vi "ControlGenerator_Main.vi"() -> ()   [LabVIEW 2014]
uses:
  <vilib>/LabVIEW Icon API/LabVIEW Icon API.lvlib
  <vilib>/LabVIEW Icon API/lv_icon/Classes/Icon/Icon.lvclass
  controls/CC_TypeSelectionEnum.ctl
  controls/CC_CreateNewCTLSettings.ctl
  <vilib>/Utility/miscctls.llb/LVPointTypeDef.ctl
  <vilib>/Utility/file.llb/Read Delimited Spreadsheet (string).vi
panel:
  in  "Stop":bool
  in  "PLM_Tab Control":enum32{"Overview", "Batch"}(tab)
  in  "ShowNewCTL?":bool=TRUE
  in  "AppendNewDataToControl?":enum32{"discard", "top", "bottom"}(radio)=enum."top" caption="append new data to control?"
  in  "RowCol_index_ForRing":i32=1 caption="# index for\nthe values" min=0 step=1
  in  "Save control to file?":bool
  in  "ignore empty fields?":bool
  in  "RowCol_index_All":i32 caption="# index\nfor the text" min=0 step=1
  in  "CreateSingleControl":bool
  in  "Clipboard Data":string[][](array[string])
  in  "GetClipboardData":bool
  in  "Select the new type":T1=enum."Enum"
  in  "Row or Col?":enum32{"Row", "Column"}(radio) caption="which axis?"
  in  "Single Control Save Path":path=path "C:/Program Files/National Instruments/MyProjects/functions/Scripting/Controls/dummy_output/abc.ctl" caption="Save Path"
  in  "file format (%.3f, %s, %d)":string="%.3f"
  in  "delimiter ('\\t', '\\s', ',')":string="\\t"
  out "Batch_Status":string
  in  "Batch_RowCol_index_ForRing":i32=1 caption="# index for\nthe values" min=0 step=1
  in  "Batch_ignore empty fields?":bool=TRUE caption="ignore empty entries?"
  in  "Batch_RowCol_index_All":i32 caption="# index\nfor the text" min=0 step=1
  in  "BatchSelect the new type":T1=enum."Enum" caption="Select the new type"
  in  "Batch_Row or Col?":enum32{"Row", "Column"}(radio)=enum."Column" caption="which axis?"
  in  "NewCTL_Open?":bool=TRUE
  in  "NewCTLFile_AddSuffix?":bool
  in  "NewCTLFile_AddPrefix?":bool
  in  "Filename of new control":enum32{"unchanged", "custom name"}(radio)
  in  "Batch_NewCTL_custom name":string caption="new name (name will be appended with an increasing number)"
  in  "suffix":string
  in  "Batch_OutputFolder":path=path "C:/Program Files/National Instruments/MyProjects/functions/Scripting/Controls/dummy_output" caption="select the output folder"
  in  "prefix":string
  in  "Palette_Save":bool
  in  "Batch_InputFolder":path=path "C:/Program Files/National Instruments/MyProjects/Board1/Lists" caption="folder with textfiles (.csv, .txt, ...)"
  # "Create a single control from clipboard"
  # "Create controls from files"
  # "Note: Ring and Comboboxes are not automatically enumerated.\nTherefore you must provide a row or column with unique entries.\nSet this column in \"# index for the values\"."
  # "Note: if you are not happy with the results do NOT delete the output files or folder,\njust run the script with different settings again; otherwise LabVIEW will complain \nabout having two controls with the same name in memory"
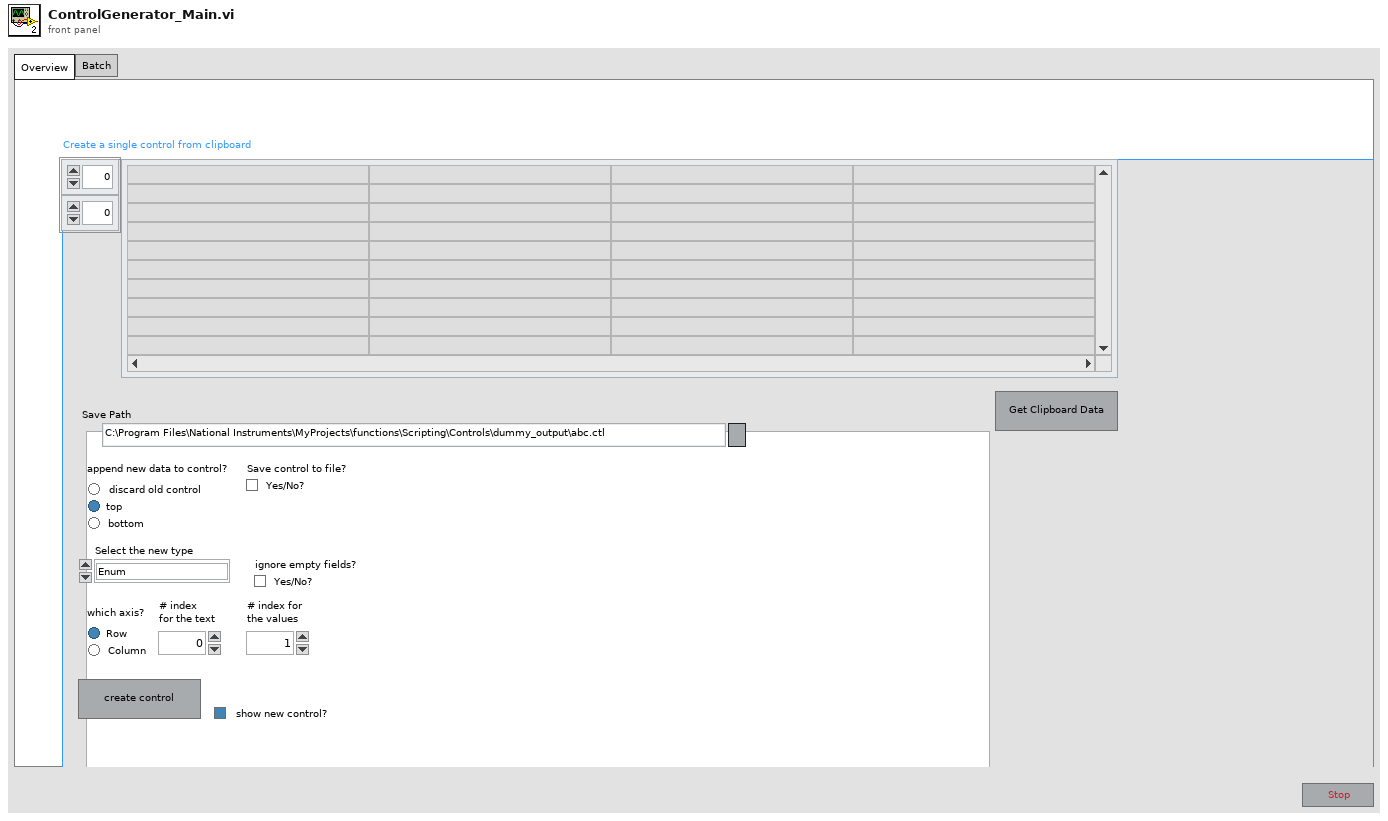
[diagram p1: front panel]
types:
  T1 = typedef "CC_TypeSelectionEnum.ctl" = enum16{"Array", "Enum", "Ring", "Text Combobox"}
  T2 = cluster{"ShowCurrentEventFrame?":bool, "IgnoreTimeoutCase?":bool}
  T3 = cluster{"VI_SM_CS_Name (In)":string, "VI_SM_CS_Name (In)":string, "Debug Mode? (F)":bool, "EventStructureDebugOptions":cluster{"ShowCurrentEventFrame?":bool, "IgnoreTimeoutCase?":bool}}
  T4 = enum8{"Enabled", "Disabled", "Disabled and Grayed Out"}
  T5 = enum32{"invalid app kind", "Development System", "Run Time System", "Student Edition", "Embedded LabVIEW", "Evaluation", "Custom"}
  T6 = typedef "LVPointTypeDef.ctl" = cluster{"Horizontal":i16, "Vertical":i16}
  T7 = enum32{"Invalid", "Standard", "Closed", "Hidden", "Minimized", "Maximized"}
  T8 = typedef "CC_CreateNewCTLSettings.ctl" = cluster{"Save control to file?":bool, "ignore empty fields?":bool, "# index\nfor the text":i32, "# index for\nthe values":i32, "Select the new type":T1, "which axis?":enum32{"Row", "Column"}, "append new data to control?":enum32{"discard", "top", "bottom"}, "open new control?":bool}
  T9 = cluster{"Core":cluster{"Current VI Reference":refnum<vi>, "Close Panel on Exit?":bool}, "CurrentItemHasModifications?":bool, "Your string data":string}
  T10 = cluster{"Current VI Reference":refnum<vi>, "Close Panel on Exit?":bool}
  T11 = typedef "imagedata.ctl" = cluster{"image type":i32, "image depth":i32, "image":u8[], "mask":u8[], "colors":u32[], "Rectangle":cluster{"left":i16, "top":i16, "right":i16, "bottom":i16}}
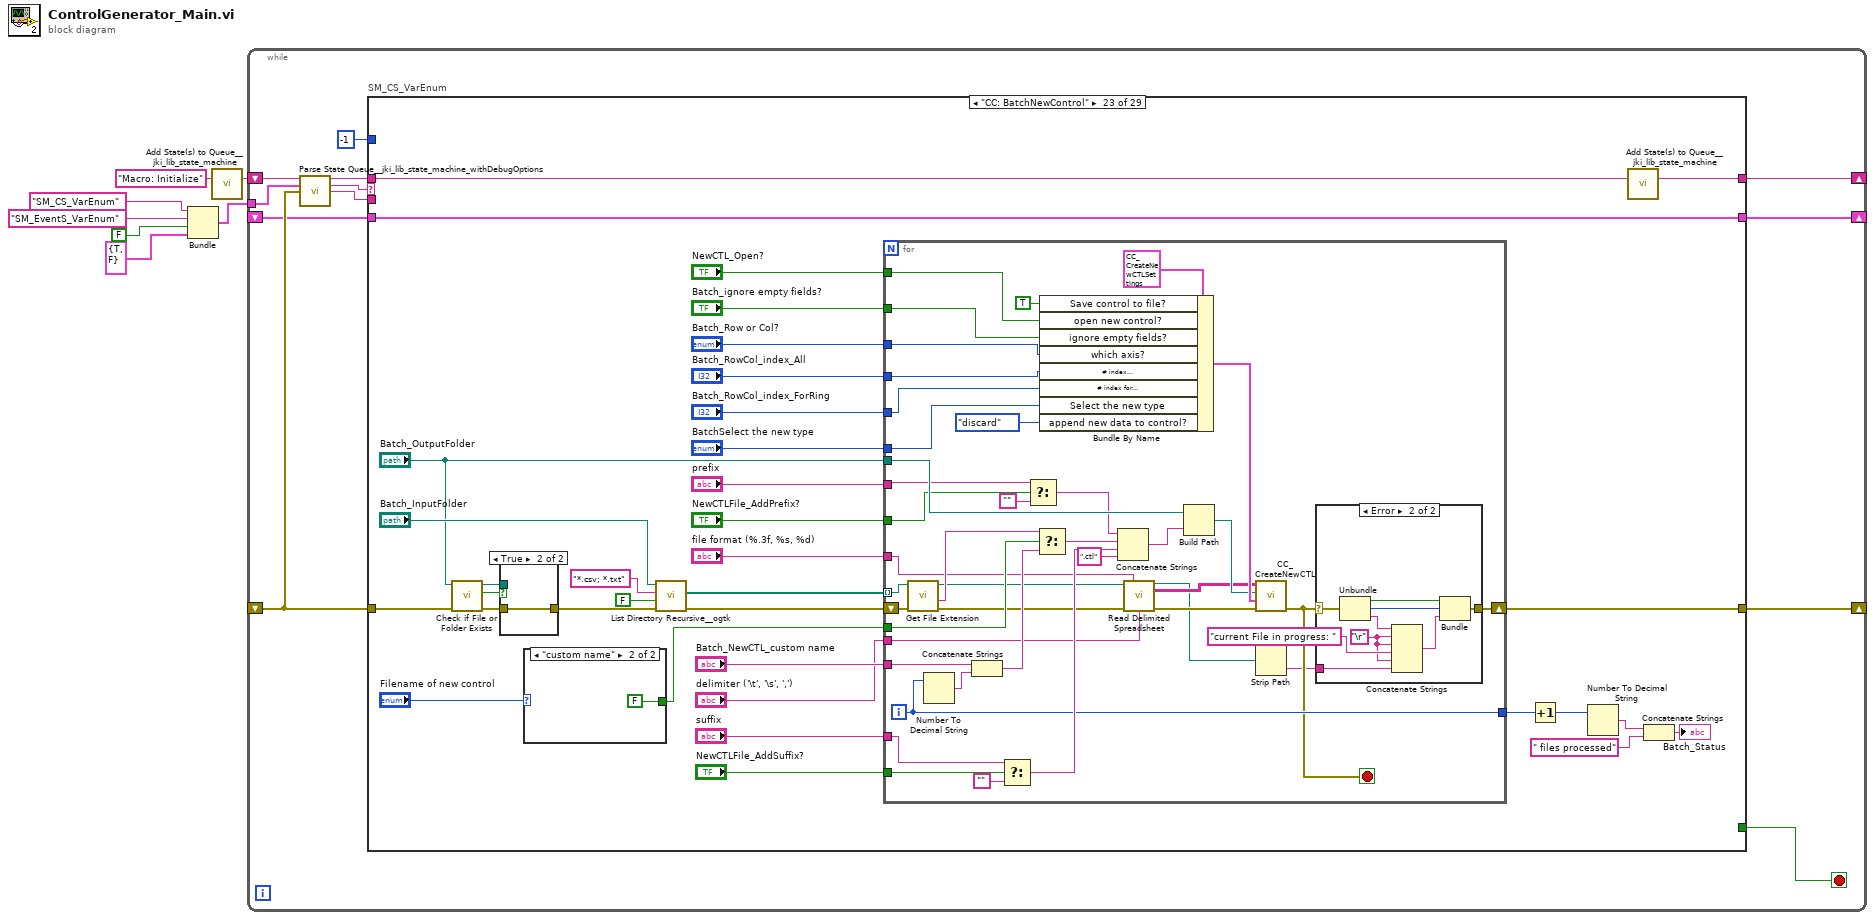
[diagram p0: block diagram]
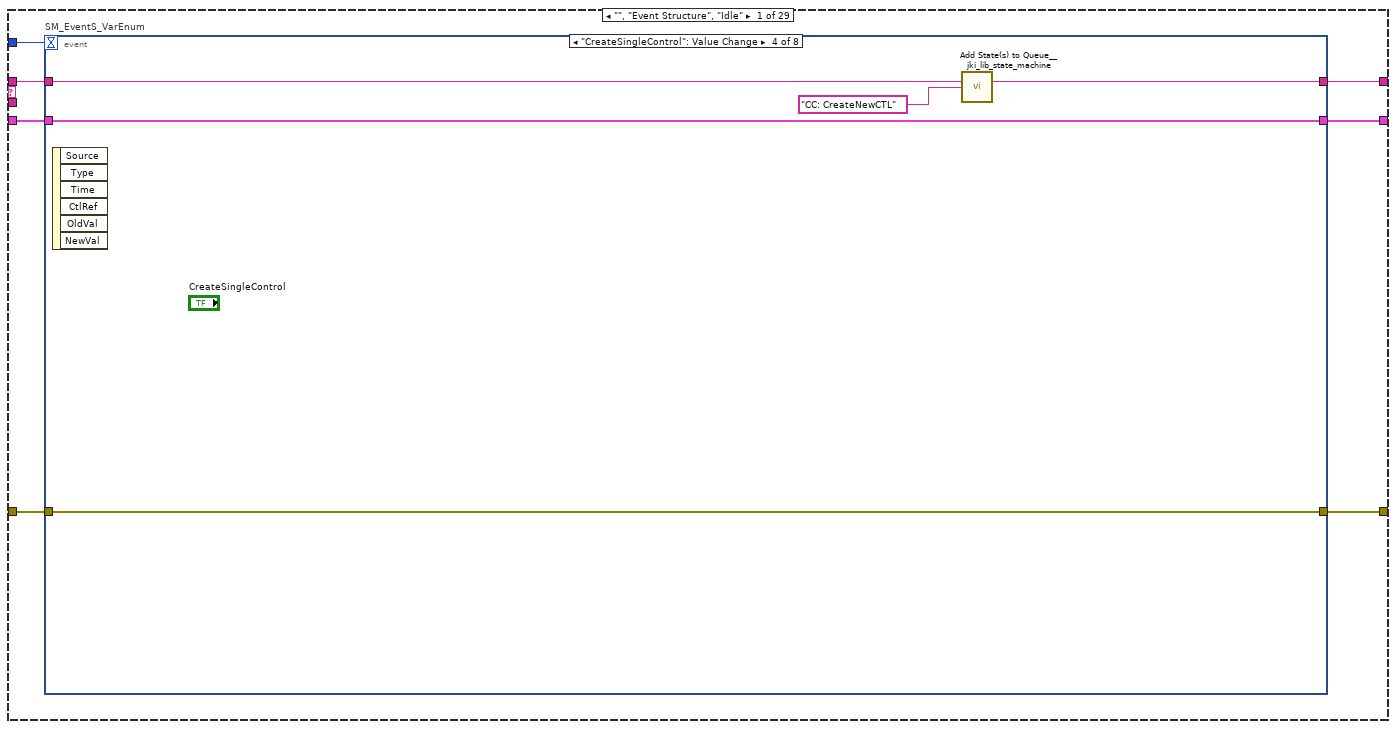
[diagram p2: hidden frame]
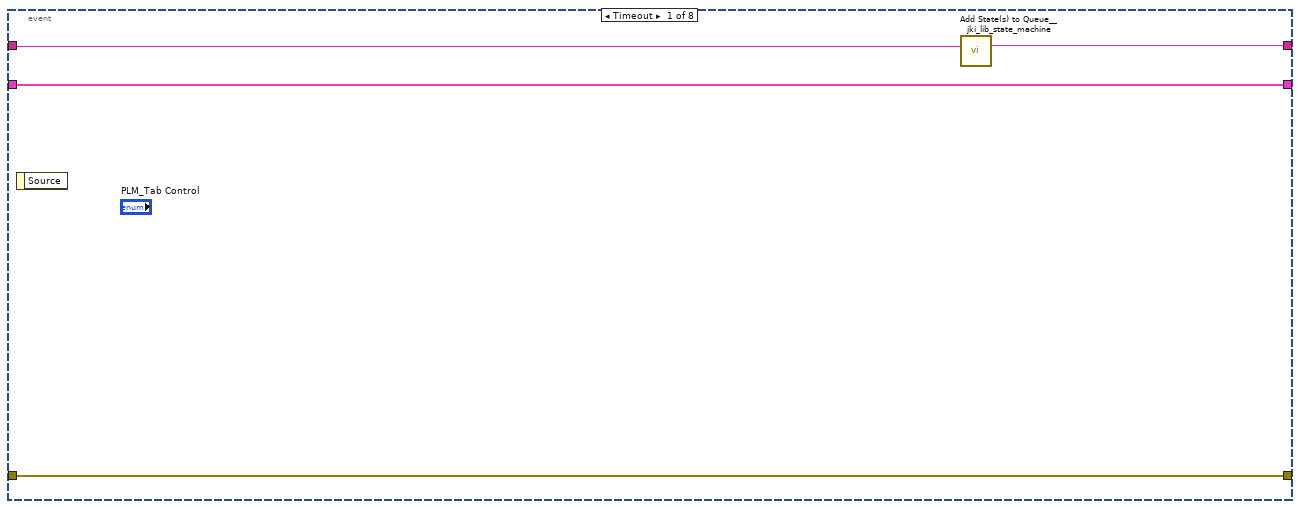
[diagram p3: hidden frame]
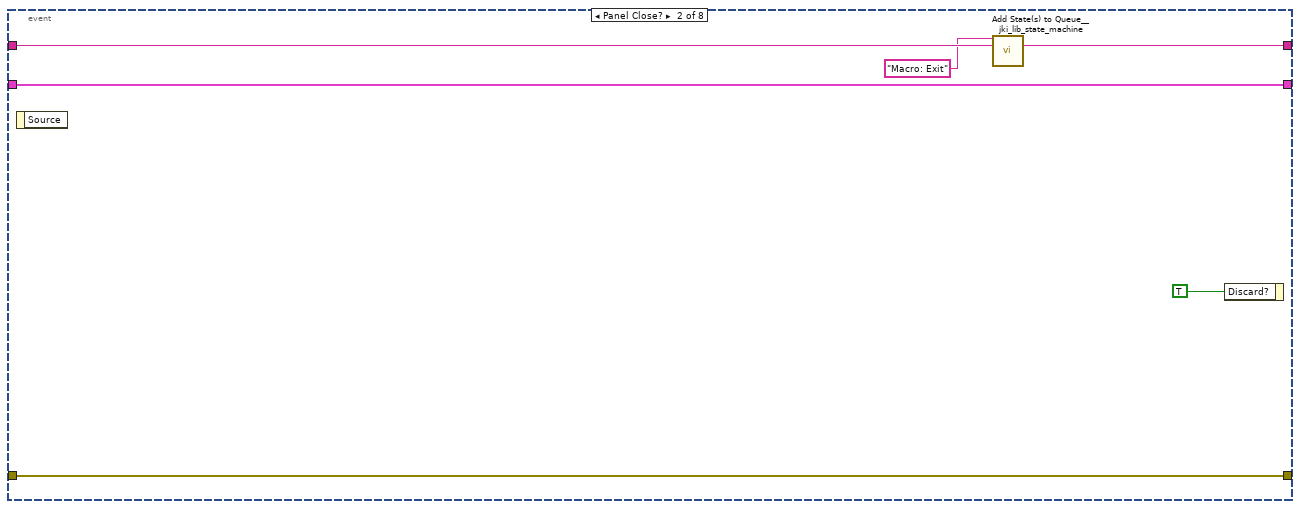
[diagram p4: hidden frame]
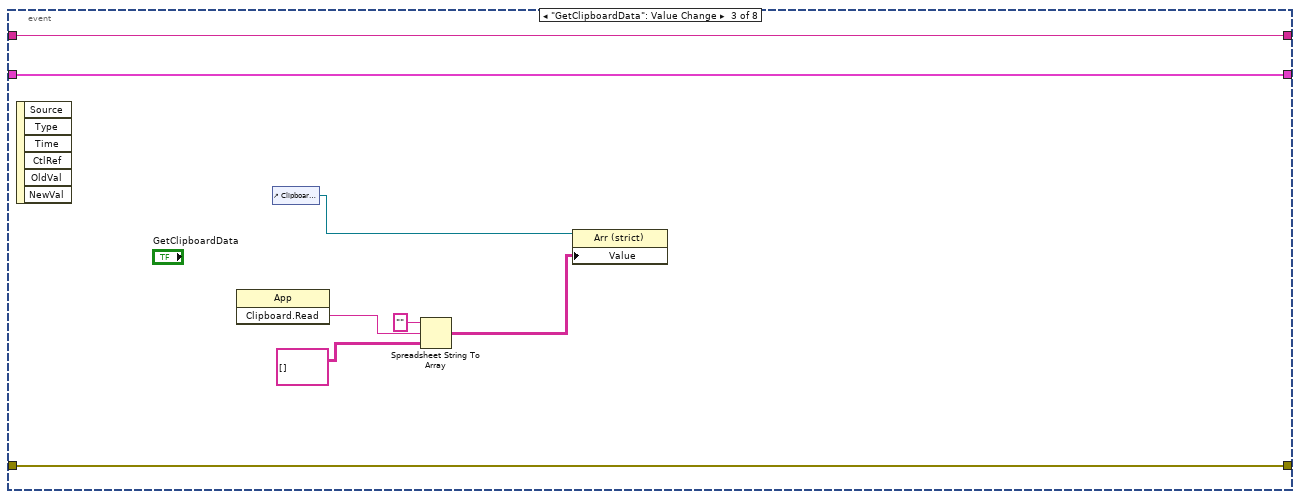
[diagram p5: hidden frame]
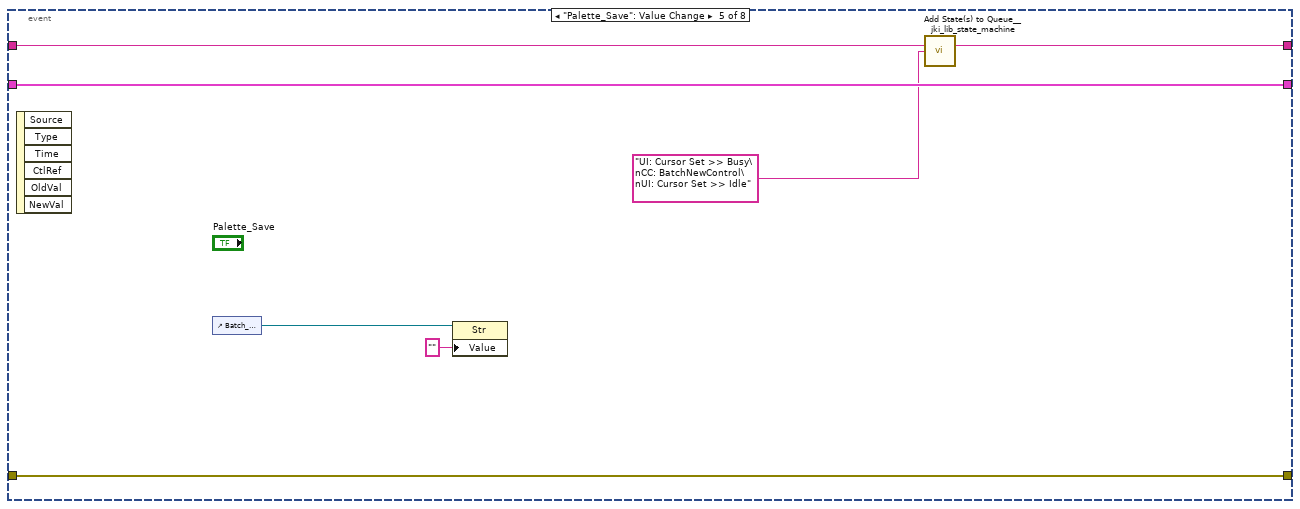
[diagram p6: hidden frame]
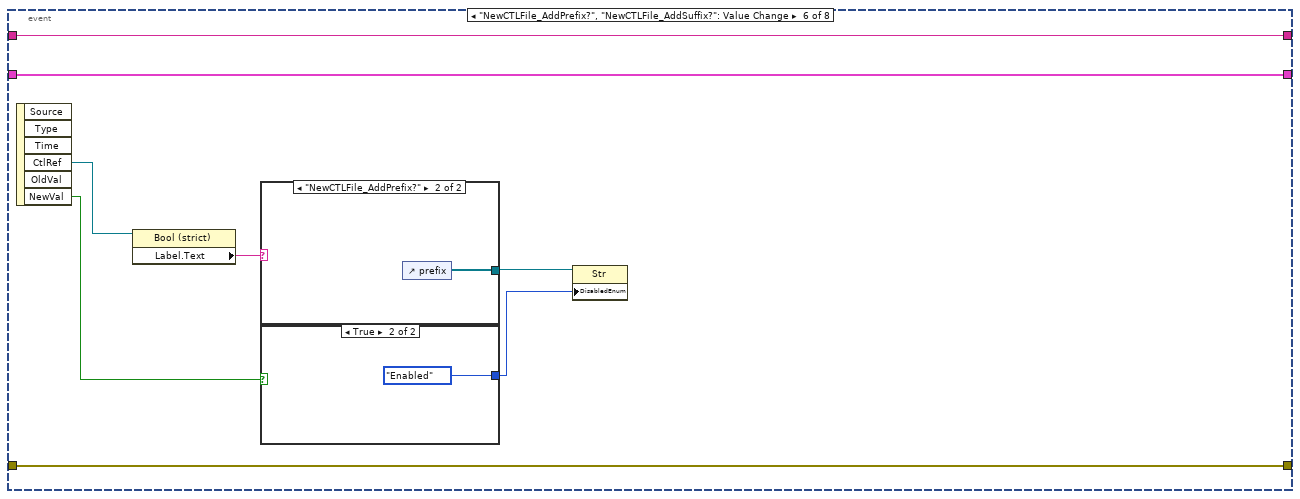
[diagram p7: hidden frame]
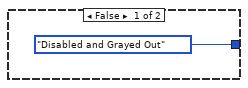
[diagram p8: hidden frame]
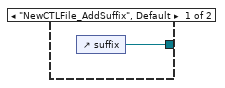
[diagram p9: hidden frame]
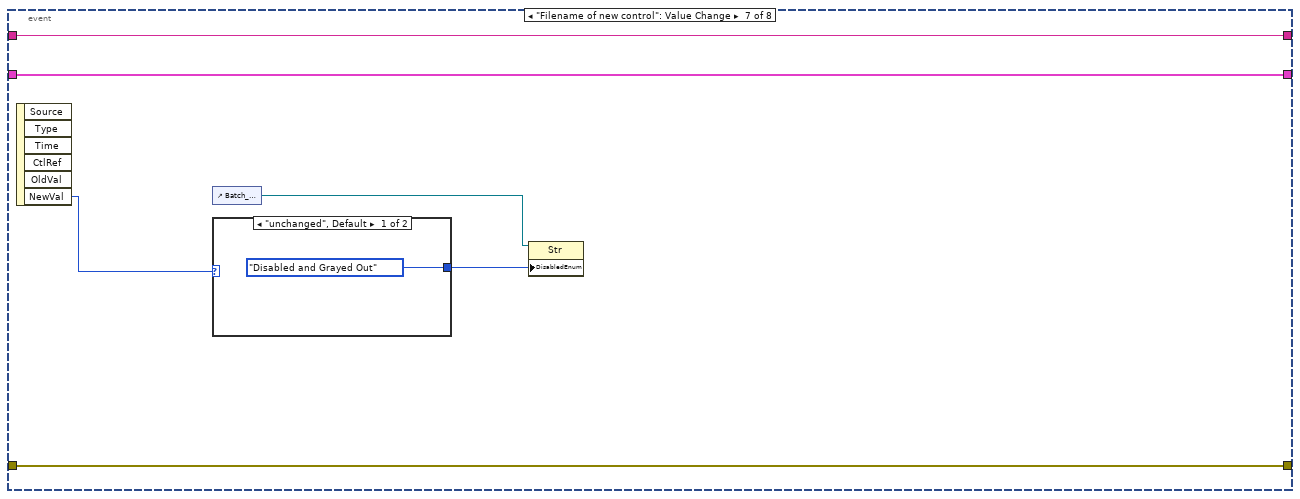
[diagram p10: hidden frame]
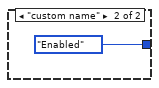
[diagram p11: hidden frame]
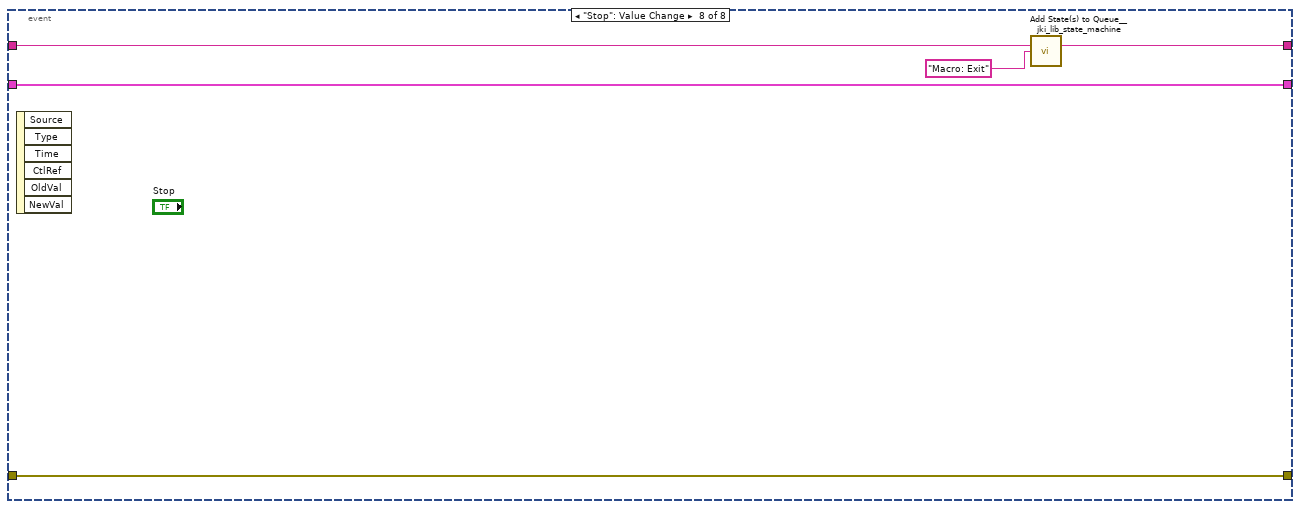
[diagram p12: hidden frame]
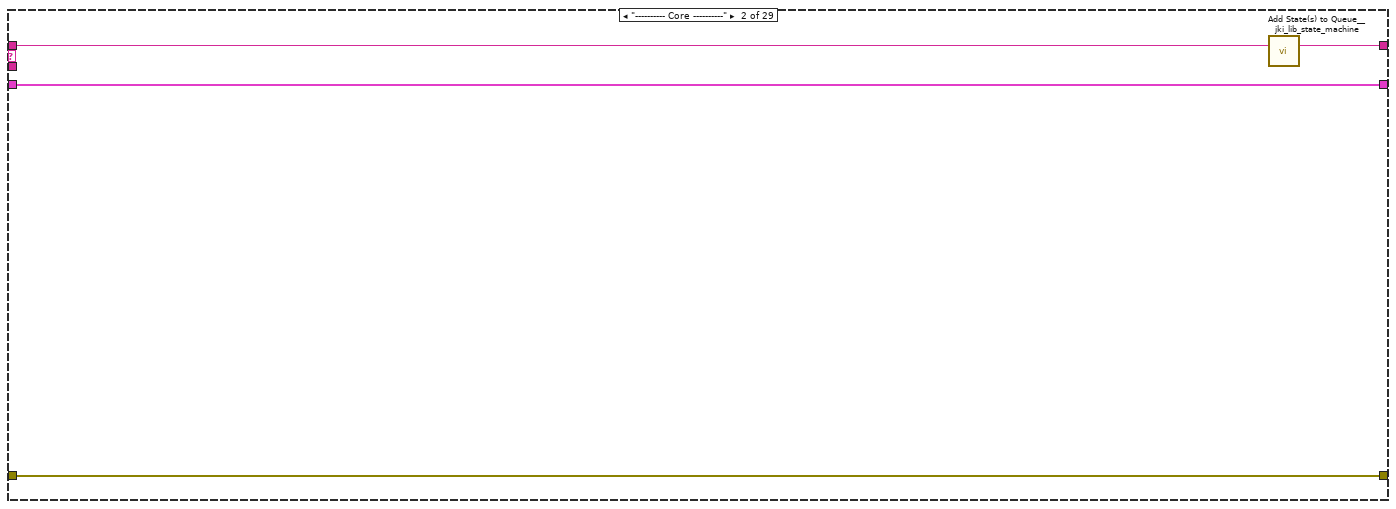
[diagram p13: hidden frame]
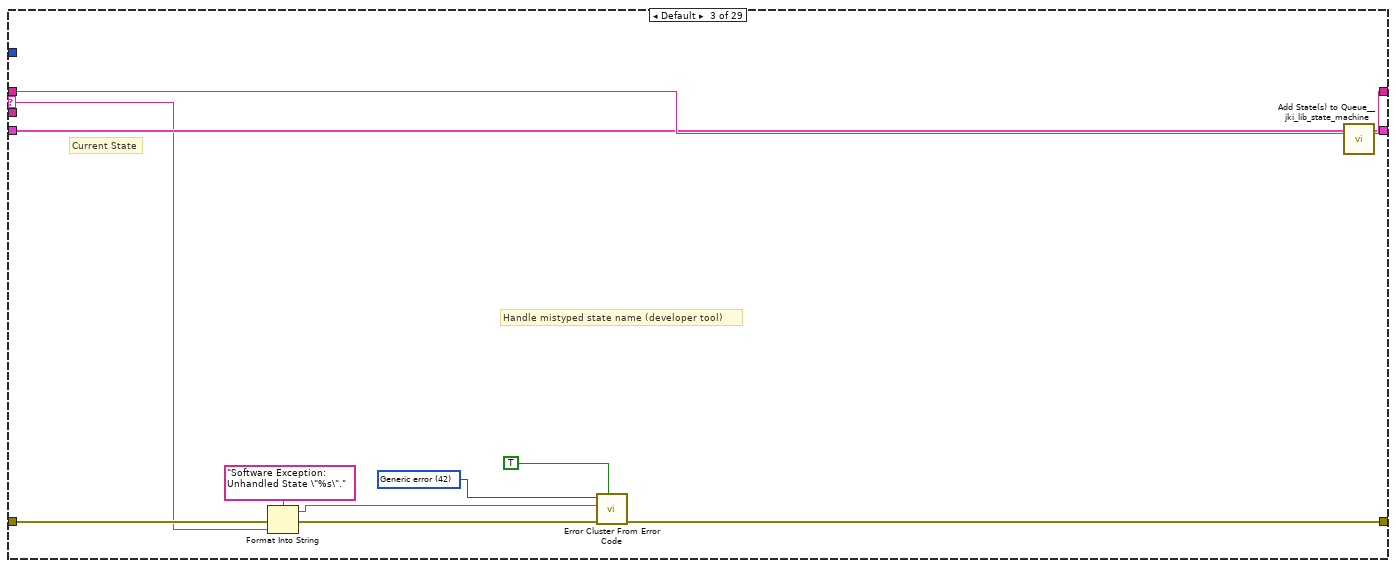
[diagram p14: hidden frame]
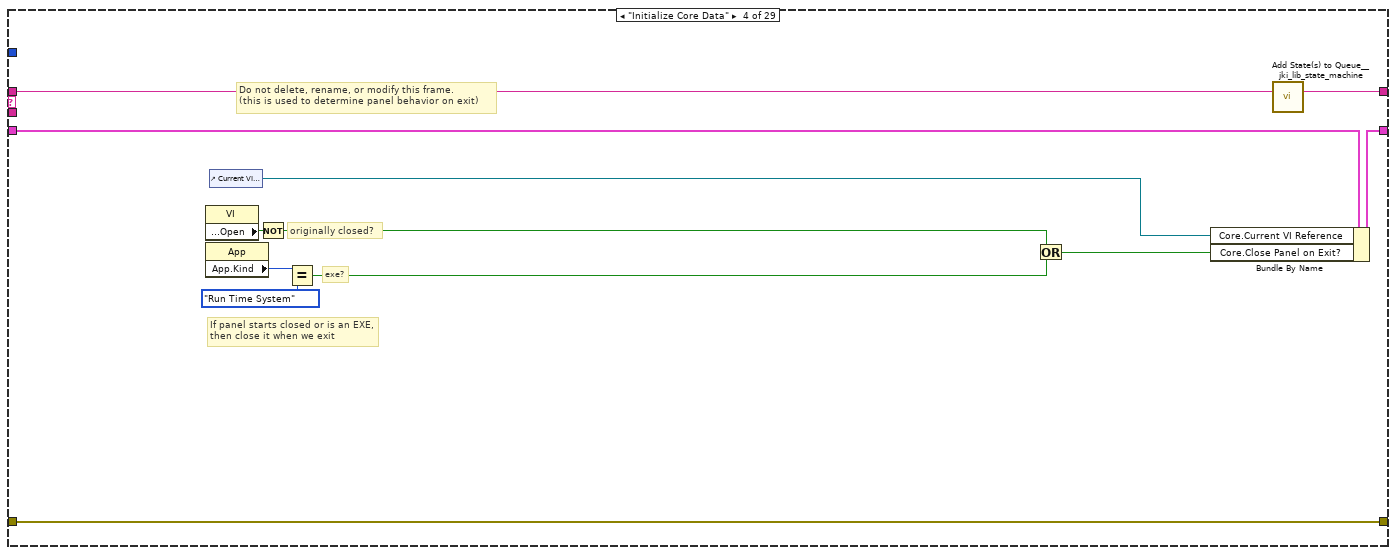
[diagram p15: hidden frame]
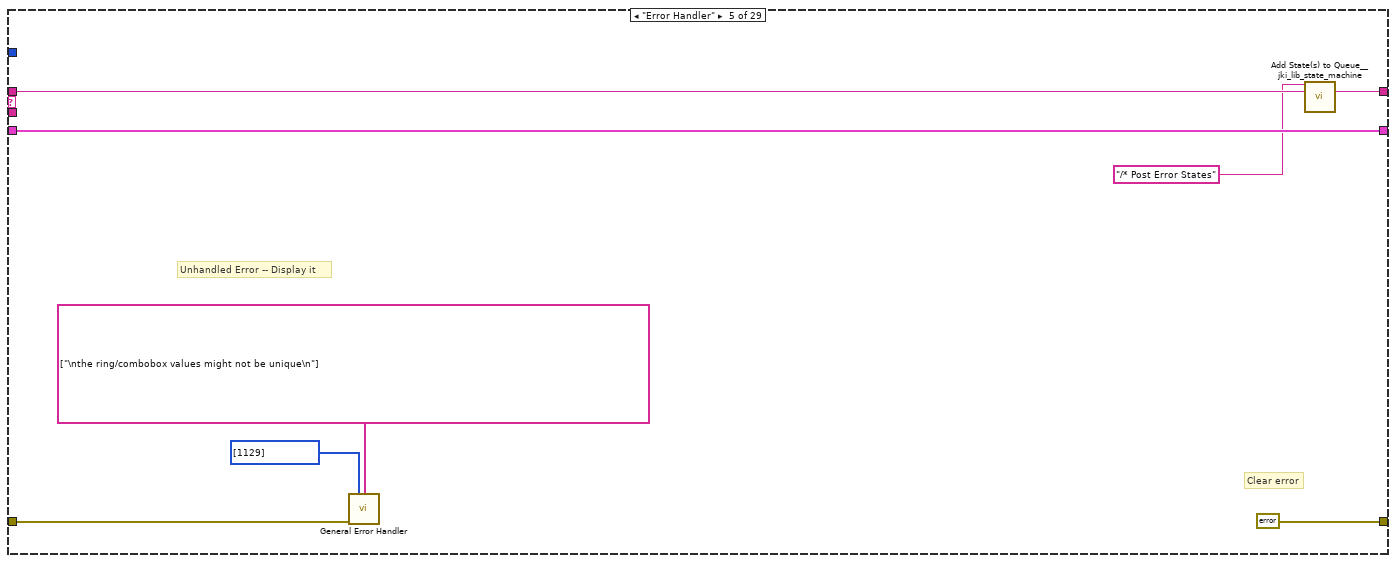
[diagram p16: hidden frame]
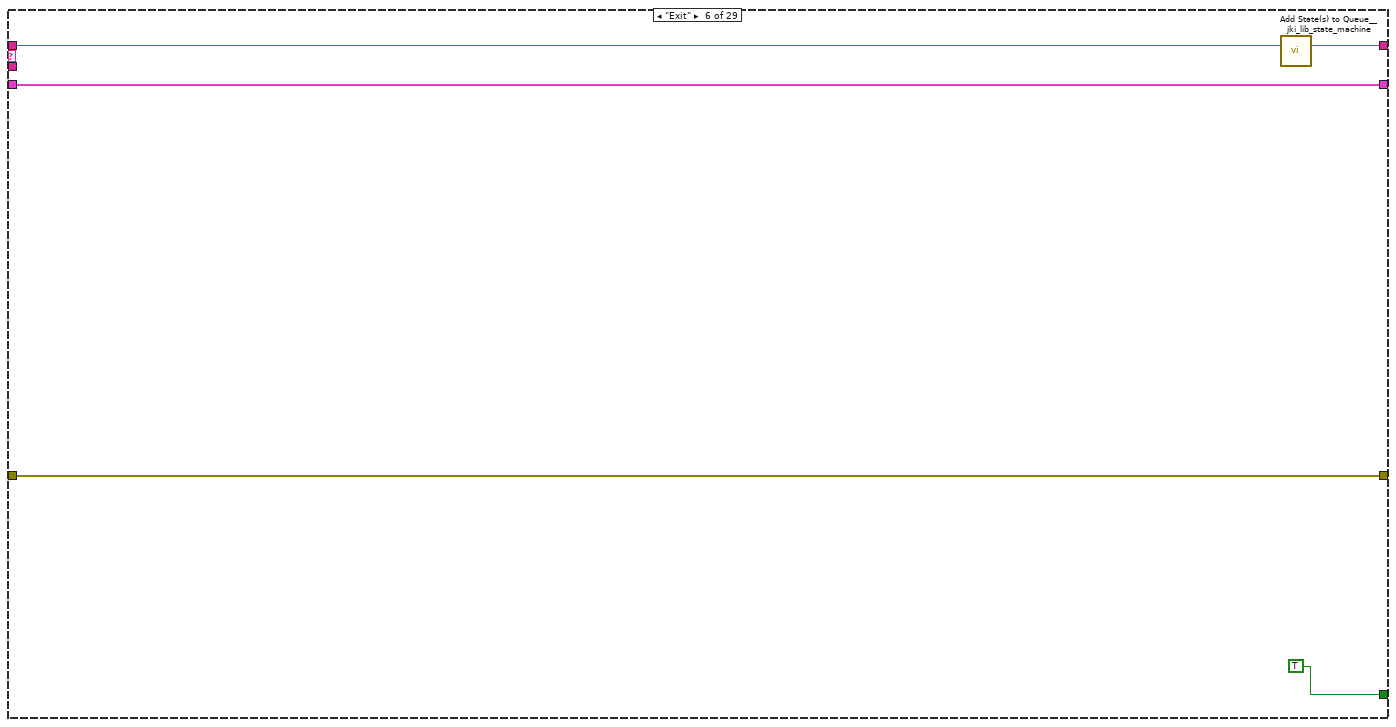
[diagram p17: hidden frame]
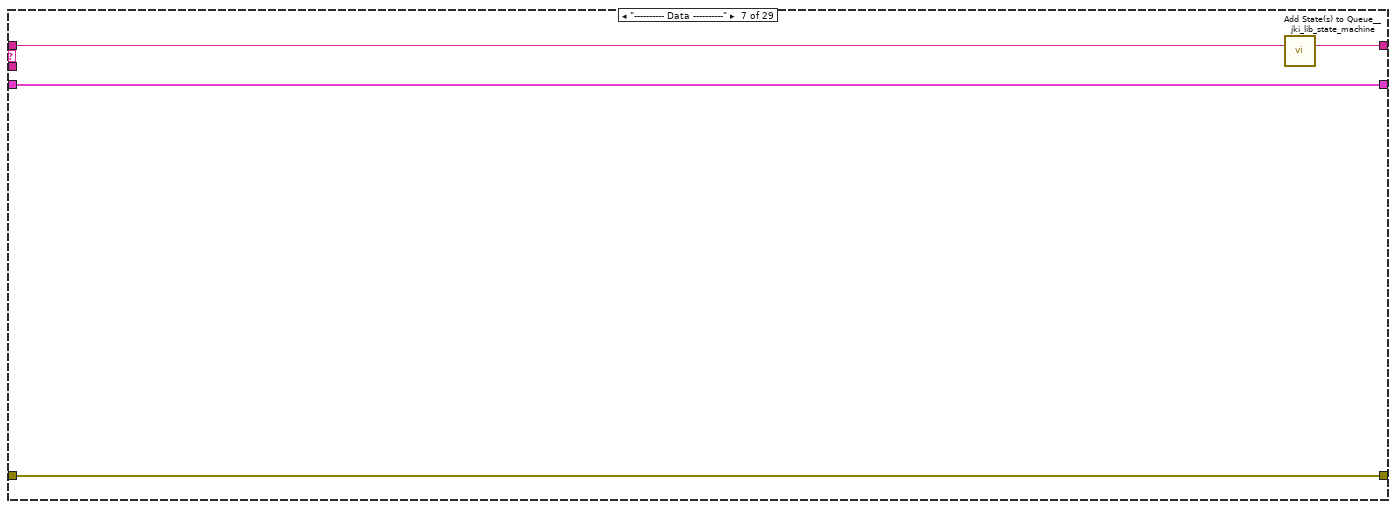
[diagram p18: hidden frame]
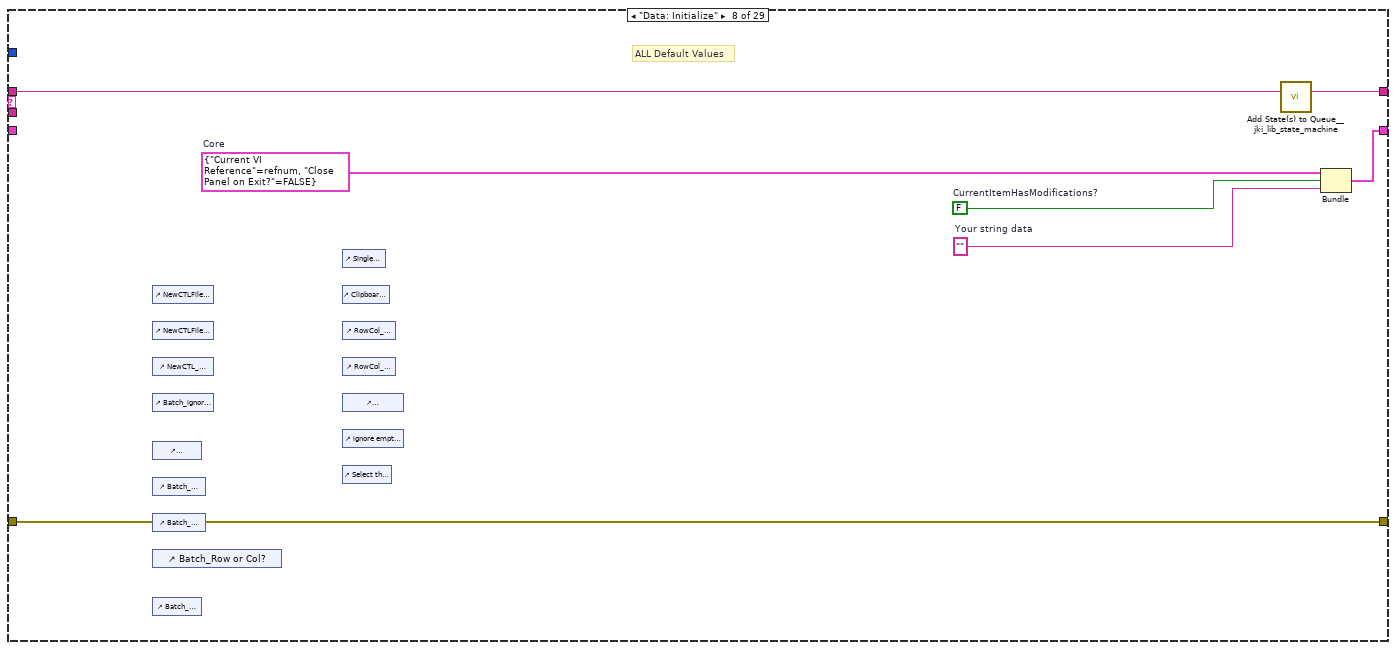
[diagram p19: hidden frame]
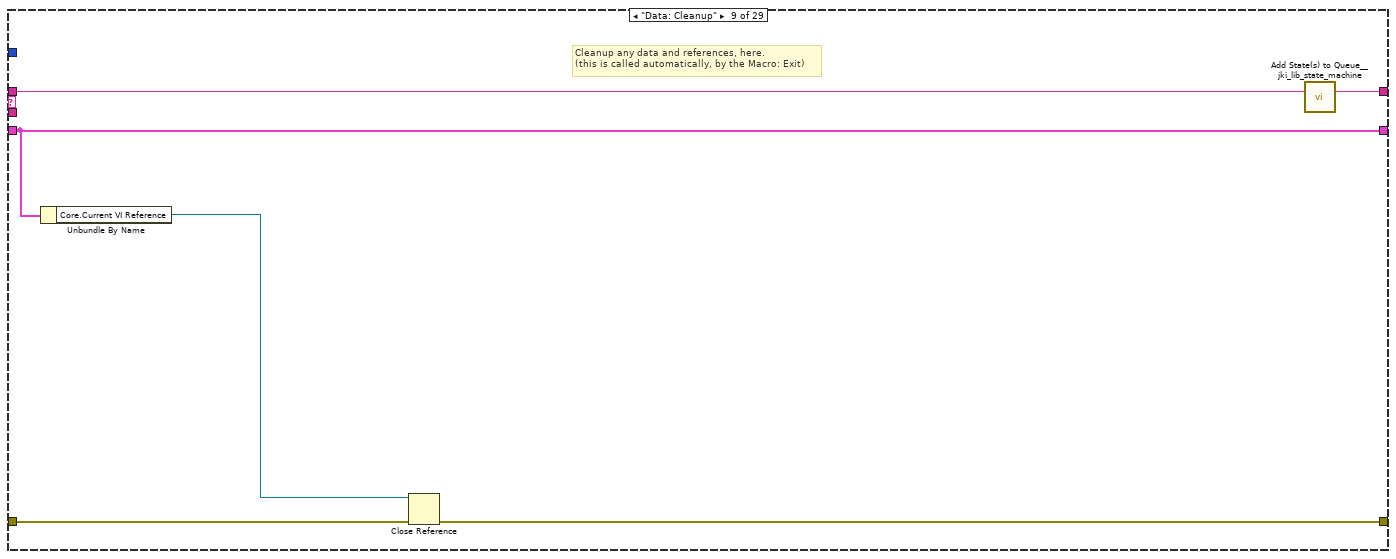
[diagram p20: hidden frame]
diagram:
  n1 = Bundle("VI_SM_CS_Name (In)"="SM_CS_VarEnum", "VI_SM_CS_Name (In)"="SM_EventS_VarEnum", "Debug Mode? (F)"=FALSE, "EventStructureDebugOptions"=T2 {"ShowCurrentEventFrame?"=TRUE, "IgnoreTimeoutCase?"=FALSE}) -> (w5:T3)  [unwired: 1 in]
  n2 = call <vilib>:"Add State(s) to Queue__jki_lib_state_machine.vi"("State(s) in (\"\")"="Macro: Initialize") -> ("States Out"=w6:string)  [unwired: 14 in]
  n3 = while {
    shift-right: [w11] -> _
    shift-left: _ -> [w10]
    shift-right: [w14] -> _
    shift-left: _ -> [w19]
    shift-right: [w13] -> _
    shift-left: w6 -> [w15]
    tunnel: w5 -> [w8]
    stop <- w12 stop-if-true
    n4 = call "Parse State Queue__jki_lib_state_machine_withDebugOptions.vi"("State Queue"=w15, "SM_StateFollower_UserSettings"=w8, "Error In (no error)"=w19) -> ("Remaining States"=w17:string, "Current State"=w18:string, "Arguments"=w16:string)  [unwired: 10 in]
    n5 = case "SM_CS_VarEnum" shown="\"CC: BatchNewControl\"" w18 {
      selector: w18 -> [_ _ w86 _ _ _ _ _ _ _ _ _ _ _ _ _ _ _ _ _ _ _ _ _ _ _ _ _ _]
      tunnel: w17 -> [w26 w85 w90 w108 w116 w121 w125 w132 w138 w142 w151 w155 w160 w168 w180 w191 w217 w222 w232 w236 w240 w257 w292 w351 w354 w366 w380 w390 w395]
      tunnel: w16 -> [_ _ _ _ _ _ _ _ _ _ _ _ _ w163 w177 w185 _ _ _ _ _ _ _ _ _ _ _ _ _]
      tunnel: w10 -> [w24 w82 w88 w99 w113 w119 w122 _ w133 w139 w148 w153 w158 w166 w176 w187 w214 w219 w229 w233 w238 w255 w289 w350 w363 w371 w384 w388 w393]
      tunnel: [w23 w83 w92 w105 errorcluster {"status"=FALSE, "code"=0, "source"=""} ("error out") w118 w123 w129 w134 w140 w149 w152 w157 w164 w175 w188 w215 w220 w230 w234 w237 w250 w290 w352 w361 w370 w382 w392 w394] -> w14
      tunnel: w19 -> [w22 w83 w91 w105 w112 w118 w123 w129 w135 w140 w149 w152 w157 w165 w178 w189 w215 w220 w230 w234 w237 w249 w270 w352 w360 w369 w382 w392 w394]
      tunnel: [w25 w84 w89 w107 w115 w120 w124 w131 w137 w141 w150 w154 w159 w167 w179 w190 w216 w221 w231 w235 w239 w256 w291 w351 w355 w367 w381 w391 w395] -> w13
      tunnel: [_ _ _ _ _ TRUE _ _ _ _ _ _ _ _ _ _ _ _ _ _ _ _ _ _ _ _ _ _ _] -> w12
      tunnel: [w21 w82 w88 w106 w113 w119 w122 w130 w133 w139 w148 w153 w158 w166 w176 w187 w214 w219 w229 w233 w238 w255 w289 w350 w363 w371 w383 w388 w393] -> w11
      tunnel: -1 ("Timeout") -> [w20 _ _ _ _ _ _ _ _ _ _ _ _ _ _ _ _ _ _ _ _ _ _ _ _ _ _ _ _]
      frame "", "Event Structure", "Idle" {
        n6 = event "SM_EventS_VarEnum" shown="[3] \"CreateSingleControl\": Value Change" {
          selector: _ -> [_ _ _ _ _ _ _ _]
          dyn-events: _ -> [_ _ _ _ _ _ _ _]
          timeout: w20 -> [_ _ _ _ _ _ _ _]
          tunnel: w26 -> [w30 w36 w42 w46 w53 w64 w74 w78]
          tunnel: [w29 w35 w42 w47 w54 w64 w74 w79] -> w25
          tunnel: w24 -> [w27 w33 w43 w48 w55 w62 w72 w81]
          tunnel: [w28 w34 w44 w49 w56 w63 w73 w80] -> w23
          tunnel: w22 -> [w28 w34 w44 w49 w56 w63 w73 w80]
          tunnel: [w27 w33 w43 w48 w55 w62 w72 w81] -> w21
          event Timeout {
            n7 = event-data() -> ()  [unwired: 1 in, 1 out]
            n8 = call <vilib>:"Add State(s) to Queue__jki_lib_state_machine.vi"("State(s) in (\"\")"=w30) -> ("States Out"=w29:string)  [unwired: 14 in]
          }
          event Panel Close? {
            n9 = event-data() -> ()  [unwired: 1 in, 1 out]
            n10 = call <vilib>:"Add State(s) to Queue__jki_lib_state_machine.vi"("State(s) in Front (\"\")"="Macro: Exit", "State(s) in (\"\")"=w36) -> ("States Out"=w35:string)  [unwired: 13 in]
            n11 = event-data("Discard?"=TRUE) -> ()  [unwired: 1 in, 1 out]
          }
          event "GetClipboardData": Value Change {
            n12 = event-data() -> ()  [unwired: 1 in, 6 out]
            n13 = invoke class="App" method="Clipboard.Read"() -> ("Read Clipbrd"=w38:string)  [unwired: 3 in, 2 out]
            n14 = control-ref of="Clipboard Data"() -> (w41:refnum<vi>)
            n15 = Spreadsheet String To Array(format string="", spreadsheet string=w38, array type (2D Dbl)=string[][] [] ("Value")) -> (array=w39:string[][])  [unwired: 1 in]
            n16 = property class="Arr (strict)"(reference=w41, "Value"=w39) -> ()  [unwired: 1 in, 2 out]
          }
          event "CreateSingleControl": Value Change {
            n17 = event-data() -> ()  [unwired: 1 in, 6 out]
            n18 = call <vilib>:"Add State(s) to Queue__jki_lib_state_machine.vi"("State(s) in (\"\")"=w46, "State(s) at Back (\"\")"="CC: CreateNewCTL" ("State(s) at Back (\"\")")) -> ("States Out"=w47:string)  [unwired: 13 in]
          }
          event "Palette_Save": Value Change {
            n19 = event-data() -> ()  [unwired: 1 in, 6 out]
            n20 = control-ref of="Batch_Status"() -> (w51:refnum<vi>)
            n21 = property class="Str"(reference=w51, "Value"="") -> ()  [unwired: 1 in, 2 out]
            n22 = call <vilib>:"Add State(s) to Queue__jki_lib_state_machine.vi"("State(s) in (\"\")"=w53, "State(s) at Back (\"\")"="UI: Cursor Set >> Busy\nCC: BatchNewControl\nUI: Cursor Set >> Idle") -> ("States Out"=w54:string)  [unwired: 13 in]
          }
          event "NewCTLFile_AddPrefix?", "NewCTLFile_AddSuffix?": Value Change {
            n23 = event-data() -> ("CtlRef"=w60:refnum<vi>, "NewVal"=w57:bool)  [unwired: 1 in, 4 out]
            n24 = property class="Bool (strict)"(reference=w60) -> ("Label.Text"=w59:string)  [unwired: 1 in, 2 out]
            n25 = case shown="\"NewCTLFile_AddPrefix?\"" w59 {
              tunnel: [w67 w68] -> w61
              frame "NewCTLFile_AddSuffix", Default {
                n26 = control-ref of="suffix"() -> (w67:refnum<vi>)
              }
              frame "NewCTLFile_AddPrefix?" {
                n27 = control-ref of="prefix"() -> (w68:refnum<vi>)
              }
            }
            n28 = case shown="True" w57 {
              tunnel: [T4."Disabled and Grayed Out" ("Disabled") T4."Enabled" ("Disabled")] -> w58
              frame False {
              }
              frame True {
              }
            }
            n29 = property class="Str"(reference=w61, "DisabledEnum"=w58) -> ()  [unwired: 1 in, 2 out]
          }
          event "Filename of new control": Value Change {
            n30 = event-data() -> ("NewVal"=w71:enum32{"unchanged", "custom name"})  [unwired: 1 in, 5 out]
            n31 = control-ref of="Batch_NewCTL_custom name"() -> (w69:refnum<vi>)
            n32 = case shown="\"unchanged\", Default" w71 {
              tunnel: [T4."Disabled and Grayed Out" ("Disabled") T4."Enabled" ("Disabled")] -> w70
              frame "unchanged", Default {
              }
              frame "custom name" {
              }
            }
            n33 = property class="Str"(reference=w69, "DisabledEnum"=w70) -> ()  [unwired: 1 in, 2 out]
          }
          event "Stop": Value Change {
            n34 = event-data() -> ()  [unwired: 1 in, 6 out]
            n35 = call <vilib>:"Add State(s) to Queue__jki_lib_state_machine.vi"("State(s) in (\"\")"=w78, "State(s) at Back (\"\")"="Macro: Exit") -> ("States Out"=w79:string)  [unwired: 13 in]
          }
        }
      }
      frame "---------- Core ----------" {
        n36 = call <vilib>:"Add State(s) to Queue__jki_lib_state_machine.vi"("State(s) in (\"\")"=w85) -> ("States Out"=w84:string)  [unwired: 14 in]
      }
      frame Default {
        w95 = 42 items=["No error", "Argument error", "Memory is full", "Out of zone", "End of file", "File already open", "Generic file I/O error", "File not found", "File permission error", "Disk is full", "Duplicate path", "Too many files open", "System feature not enabled", "Resource file not found", "Cannot add resource", "Resource not found", "Image not found", "Image memory error", "Pen does not exist", "Config type invalid", "Config token not found", "Config parse error", "Config memory error", "Bad external code format", "Bad external code offset", "External code not present", "Null window", "Destroy window error", "Null menu", "Print aborted", "Bad print record", "Print driver error", "Windows error during printing", "Memory error during printing", "Print dialog error", "Generic print error", "Invalid device refnum", "Device not found", "Device parameter error", "Device unit error", "Cannot open device", "Device call aborted", "Generic error", "Cancelled by user", "Object ID too low", "Object ID too high", "Object not in heap", "Unknown heap", "Unknown object (invalid DefProc)", "Unknown object (DefProc not in table)", "Message out of range", "Invalid (null) method", "Unknown message", "Manager call not supported", "Bad address", "Network operation in progress", "Network operation timed out", "Connection is busy", "Network attribute not supported", "Network error", "Address in use", "System out of memory", "Connection aborted", "Connection refused", "Not connected", "Already connected", "Connection closed", "Initialization error (interapplication manager)", "Bad occurrence", "Wait on unbound occurrence handler", "Occurrence queue overflow", "Datalog type conflict", "Unused", "Unrecognized type (interapplication manager)", "Memory corrupt", "Failed to make temporary DLL", "Old CIN version", "Drag socket not found", "Failed to load drop-object", "Failed to register OLE object", "Failed to release OLE object", "Format specifier type mismatch", "Unknown format specifier", "Too few format specifiers", "Too many format specifiers", "Scan failed", "Newer CIN version", "Error converting to variant", "Runtime menu error", "Password tampered", "Variant attribute not found", "Incompatible variant data type", "Event data is not available", "Event Store is not present", "Occurrence is not found", "Event Queue is not created", "Event info is not available", "Refnum passed is NULL", "Error retrieving Class GUID", "Error retrieving CoClass GUID", "Error retrieving TypeLib GUID.", "Bad built application magic bytes.", "Specific driver is different from the specific driver associated with the Logical Name.", "There is no session opened to the class driver.", "Max Error", "MAX - Error with config objects", "MAX - Error loading configuration", "MAX - Group not supported"]
        # "Current State"
        # "Handle mistyped state name (developer tool)"
        n37 = Format Into String(format string="Software Exception: Unhandled State \"%s\"." ("message"), error in=w91, w86) -> (resulting string=w94:string, error out=w93:errorcluster)  [unwired: 1 in]
        n38 = call <vilib>:"Error Cluster From Error Code.vi"("show call chain? (False)"=TRUE, "error in (no error)"=w93, "error message (\"\")"=w94, "error code (0)"=w95) -> ("error out"=w92:errorcluster)  [unwired: 5 in]
        n39 = call <vilib>:"Add State(s) to Queue__jki_lib_state_machine.vi"("State(s) in (\"\")"=w90) -> ("States Out"=w89:string)  [unwired: 14 in]
      }
      frame "Initialize Core Data" {
        # "Do not delete, rename, or modify this frame.\n(this is used to determine panel behavior on exit)"
        # "originally closed?"
        # "exe?"
        # "If panel starts closed or is an EXE, then close it when we exit"
        n40 = property class="VI"() -> ("Front Panel.Open"=w104:bool)  [unwired: 2 in, 2 out]
        n41 = property class="App"() -> ("App.Kind"=w103:T5)  [unwired: 2 in, 2 out]
        n42 = control-ref of="Current VI Reference"() -> (w97:refnum<vi>)
        n43 = Not(x=w104) -> (.not. x?=w101:bool)
        n44 = Equal?(x=w103, y=T5."Run Time System" ("Application:Kind")) -> (x = y?=w100:bool)
        n45 = Or(x=w101, y=w100) -> (x .or. y?=w98:bool)
        n46 = Bundle By Name(cluster=w99, "Core.Current VI Reference"=w97, "Core.Close Panel on Exit?"=w98) -> (w106:T9)
        n47 = call <vilib>:"Add State(s) to Queue__jki_lib_state_machine.vi"("State(s) in (\"\")"=w108) -> ("States Out"=w107:string)  [unwired: 14 in]
      }
      frame "Error Handler" {
        # "Unhandled Error -- Display it"
        # "Clear error"
        n48 = call <vilib>:"General Error Handler.vi"("[user-defined codes]"=i32[] [1129], "[user-defined descriptions]"=string[] ["\nthe ring/combobox values might not be unique\n"], "error in (no error)"=w112) -> ()  [unwired: 8 in, 5 out]
        n49 = call <vilib>:"Add State(s) to Queue__jki_lib_state_machine.vi"("State(s) in Front (\"\")"="/* Post Error States", "State(s) in (\"\")"=w116) -> ("States Out"=w115:string)  [unwired: 13 in]
      }
      frame "Exit" {
        n50 = call <vilib>:"Add State(s) to Queue__jki_lib_state_machine.vi"("State(s) in (\"\")"=w121) -> ("States Out"=w120:string)  [unwired: 14 in]
      }
      frame "---------- Data ----------" {
        n51 = call <vilib>:"Add State(s) to Queue__jki_lib_state_machine.vi"("State(s) in (\"\")"=w125) -> ("States Out"=w124:string)  [unwired: 14 in]
      }
      frame "Data: Initialize" {
        w126 = T10 {"Current VI Reference"=refnum, "Close Panel on Exit?"=FALSE}  # Core
        w128 = FALSE  # CurrentItemHasModifications?
        w127 = ""  # Your string data
        # "ALL Default Values"
        n52 = control-ref of="NewCTLFile_AddPrefix?"() -> ()  [unwired: 1 out]
        n53 = control-ref of="NewCTLFile_AddSuffix?"() -> ()  [unwired: 1 out]
        n54 = control-ref of="NewCTL_Open?"() -> ()  [unwired: 1 out]
        n55 = control-ref of="Batch_ignore empty fields?"() -> ()  [unwired: 1 out]
        n56 = control-ref of="BatchSelect the new type"() -> ()  [unwired: 1 out]
        n57 = control-ref of="Batch_RowCol_index_ForRing"() -> ()  [unwired: 1 out]
        n58 = control-ref of="Batch_RowCol_index_All"() -> ()  [unwired: 1 out]
        n59 = control-ref of="Batch_Row or Col?"() -> ()  [unwired: 1 out]
        n60 = control-ref of="Batch_NewCTL_custom name"() -> ()  [unwired: 1 out]
        n61 = control-ref of="Single Control Save Path"() -> ()  [unwired: 1 out]
        n62 = control-ref of="Clipboard Data"() -> ()  [unwired: 1 out]
        n63 = control-ref of="RowCol_index_All"() -> ()  [unwired: 1 out]
        n64 = control-ref of="RowCol_index_ForRing"() -> ()  [unwired: 1 out]
        n65 = control-ref of="CreateSingleControl"() -> ()  [unwired: 1 out]
        n66 = control-ref of="ignore empty fields?"() -> ()  [unwired: 1 out]
        n67 = control-ref of="Select the new type"() -> ()  [unwired: 1 out]
        n68 = call <vilib>:"Add State(s) to Queue__jki_lib_state_machine.vi"("State(s) in (\"\")"=w132) -> ("States Out"=w131:string)  [unwired: 14 in]
        n69 = Bundle("Core"=w126, "CurrentItemHasModifications?"=w128, "Your string data"=w127) -> (w130:T9)  [unwired: 1 in]
      }
      frame "Data: Cleanup" {
        # "Cleanup any data and references, here.\n(this is called automatically, by the Macro: Exit)"
        n70 = Unbundle By Name(w133) -> ("Core.Current VI Reference"=w136:refnum<vi>)
        n71 = Close Reference(reference=w136, error in (no error)=w135) -> (error out=w134:errorcluster)
        n72 = call <vilib>:"Add State(s) to Queue__jki_lib_state_machine.vi"("State(s) in (\"\")"=w138) -> ("States Out"=w137:string)  [unwired: 14 in]
      }
      frame "---------- UI ----------" {
        # "Do not put any code in this frame.\n(It is a separator no-op. You can make a copy of this frame to create a new UI frame)"
        n73 = call <vilib>:"Add State(s) to Queue__jki_lib_state_machine.vi"("State(s) in (\"\")"=w142) -> ("States Out"=w141:string)  [unwired: 14 in]
      }
      frame "UI: Initialize" {
        # "Initialize the User Interface, here.\n(this is called automatically, by the Macro: Init)"
        n74 = Unbundle By Name(w148) -> ("Core.Current VI Reference"=w147:refnum<vi>)
        n75 = property class="VI"(reference=w147) -> ("Panel"=w146:refnum<vi>)  [unwired: 1 in, 2 out]
        n76 = property class="Pnl"(reference=w146) -> ("Panes[]"=w145:refnum<vi>[])  [unwired: 1 in, 2 out]
        n77 = Index Array(array=w145) -> (element=w144:refnum<vi>)  [unwired: 1 in]
        n78 = property class="Pane"(reference=w144, "Origin"=T6 {"Horizontal"=-8, "Vertical"=-8}) -> ()  [unwired: 1 in, 2 out]
        n79 = call <vilib>:"Add State(s) to Queue__jki_lib_state_machine.vi"("State(s) in (\"\")"=w151) -> ("States Out"=w150:string)  [unwired: 14 in]
      }
      frame "UI: PaletteLoaded" {
        # "Initialize the User Interface, here.\n(this is called automatically, by the Macro: Init)"
        n80 = call <vilib>:"Add State(s) to Queue__jki_lib_state_machine.vi"("State(s) in (\"\")"=w155) -> ("States Out"=w154:string)  [unwired: 14 in]
      }
      frame "UI: PaletteReset" {
        # "load from ini"
        # "Initialize the User Interface, here.\n(this is called automatically, by the Macro: Init)"
        n81 = disable-structure shown="Disabled" {
          frame Disabled {
            n82 = control-ref of="Batch_OutputFolder"() -> (w162:refnum<vi>)
            n83 = property class="Path"(reference=w162, "Value"=path "") -> ()  [unwired: 1 in, 2 out]
          }
          frame Enabled {
          }
        }
        n84 = call <vilib>:"Add State(s) to Queue__jki_lib_state_machine.vi"("State(s) in Front (\"\")"="PLM: DrawPalImage" ("State(s) in Front (\"\")"), "State(s) in (\"\")"=w160) -> ("States Out"=w159:string)  [unwired: 13 in]
      }
      frame "UI: Cursor Set" {
        # "Argument"
        # "Set and Unset Cursor Busy.\n(Usage: \"UI: Cursor Set >> Busy|Idle\")"
        n85 = case shown="\"Idle\", Default" w163 {
          tunnel: w165 -> [w170 w172]
          tunnel: [w169 w171] -> w164
          frame "Idle", Default {
            n86 = call <vilib>:"Unset Busy.vi"("error in (no error)"=w170) -> ("error out"=w169:errorcluster)  [unwired: 10 in]
          }
          frame "Busy" {
            n87 = call <vilib>:"Set Busy.vi"("error in (no error)"=w172) -> ("error out"=w171:errorcluster)  [unwired: 9 in, 1 out]
          }
        }
        n88 = call <vilib>:"Add State(s) to Queue__jki_lib_state_machine.vi"("State(s) in (\"\")"=w168) -> ("States Out"=w167:string)  [unwired: 14 in]
      }
      frame "UI: DeferFrontpanel" {
        n89 = case shown="\"Busy\"" w177 {
          tunnel: w178 -> [w182 w183]
          tunnel: [w182 w183] -> w174
          tunnel: [FALSE ("Defer Panel Updates") TRUE ("Defer Panel Updates")] -> w173
          frame "Idle", Default {
          }
          frame "Busy" {
          }
        }
        n90 = call "VI_Defer_Panel_Update.vi"("Defer Panel Updates"=w173, "Error In"=w174) -> ("Error Out"=w175:errorcluster)  [unwired: 9 in]
        n91 = call <vilib>:"Add State(s) to Queue__jki_lib_state_machine.vi"("State(s) in (\"\")"=w180) -> ("States Out"=w179:string)  [unwired: 14 in]
      }
      frame "UI: Front Panel State" {
        # "Argument"
        # "Set Front Panel Open or Closed\n(Usage: \"UI: Front Panel State >> Open|Close\")"
        n92 = Unbundle By Name(w187) -> ("Core.Current VI Reference"=w186:refnum<vi>)
        n93 = case shown="\"Open\", Default" w185 {
          tunnel: w189 -> [w195 w208]
          tunnel: [w197 w209] -> w188
          tunnel: w186 -> [w196 w206]
          frame "Open", Default {
            n94 = property class="VI"(reference=w196, error in=w195) -> (reference out=w193:refnum<vi>, error out=w194:errorcluster, "Front Panel.Open"=w192:bool)
            n95 = case shown="False" w192 {
              tunnel: [w200 w203] -> w197
              tunnel: w194 -> [w199 w203]
              tunnel: w193 -> [w198 _]
              frame False {
                n96 = invoke class="VI" method="FP.Open"(reference=w198, error in=w199, "Activate"=TRUE, "State"=T7."Standard") -> (error out=w200:errorcluster)  [unwired: 1 in, 4 out]
              }
              frame True {
              }
            }
          }
          frame "Close" {
            n97 = property class="VI"(reference=w206, error in=w208) -> (reference out=w205:refnum<vi>, error out=w207:errorcluster, "Front Panel.Open"=w204:bool)
            n98 = case shown="True" w204 {
              tunnel: [w210 w213] -> w209
              tunnel: w207 -> [w210 w212]
              tunnel: w205 -> [_ w211]
              frame False {
              }
              frame True {
                n99 = invoke class="VI" method="FP.Close"(reference=w211, error in=w212) -> (error out=w213:errorcluster)  [unwired: 1 in, 2 out]
              }
            }
          }
        }
        n100 = call <vilib>:"Add State(s) to Queue__jki_lib_state_machine.vi"("State(s) in (\"\")"=w191) -> ("States Out"=w190:string)  [unwired: 14 in]
      }
      frame "---------- Macro ----------" {
        n101 = call <vilib>:"Add State(s) to Queue__jki_lib_state_machine.vi"("State(s) in (\"\")"=w217) -> ("States Out"=w216:string)  [unwired: 14 in]
      }
      frame "Macro: Initialize" {
        w218 = "Data: Initialize\nInitialize Core Data\nUI: DeferFrontpanel >> Busy\nUI: Initialize\nUI: PaletteLoaded >> Idle\nUI: PaletteReset\nUI: Front Panel State >> Open\nPLM: Init\nUI: DeferFrontpanel >> Idle"  # Data: Initialize Initialize Core Data UI: DeferFrontpanel >> Busy UI: Initialize UI: PaletteLoaded >> Idle UI: PaletteReset UI: Front Panel State >> Open PLM: Init UI: DeferFrontpanel >> Idle
        n102 = call <vilib>:"Add State(s) to Queue__jki_lib_state_machine.vi"("State(s) in Front (\"\")"=w218, "State(s) in (\"\")"=w222) -> ("States Out"=w221:string)  [unwired: 13 in]
      }
      frame "Macro: Exit" {
        # "Exit Macro\n(This is called once, when the VI exits)"
        n103 = Unbundle By Name(w229) -> ("Core.Close Panel on Exit?"=w228:bool)
        n104 = Select(t="UI: Front Panel State >> Close", s=w228, f="") -> (s? t:f=w225:string)
        n105 = call <vilib>:"Add State(s) to Queue__jki_lib_state_machine.vi"("State(s) in (\"\")"=w225, "State(s) at Back (\"\")"="Data: Cleanup\nExit") -> ("States Out"=w223:string)  [unwired: 13 in]
        n106 = call <vilib>:"Add State(s) to Queue__jki_lib_state_machine.vi"("State(s) in Front (\"\")"=w223, "State(s) in (\"\")"=w232) -> ("States Out"=w231:string)  [unwired: 13 in]
      }
      frame "---------- New Category ----------" {
        # "Template Separator\n(You can make a copy of, or modify, this frame)"
        n107 = call <vilib>:"Add State(s) to Queue__jki_lib_state_machine.vi"("State(s) in (\"\")"=w236) -> ("States Out"=w235:string)  [unwired: 14 in]
      }
      frame "PLM: Init" {
        n108 = call <vilib>:"Add State(s) to Queue__jki_lib_state_machine.vi"("State(s) in (\"\")"=w240) -> ("States Out"=w239:string)  [unwired: 14 in]
      }
      frame "CC: CreateNewCTL" {
        # "for TextRings values must be unique will throw an error"
        n109 = Bundle By Name(cluster=T8 {"Save control to file?"=FALSE, "ignore empty fields?"=FALSE, "# index\nfor the text"=0, "# index for\nthe values"=0, "Select the new type"=enum."Array", "which axis?"=enum."Row", "append new data to control?"=enum."discard", "open new control?"=FALSE} ("Settings"), "open new control?"="ShowNewCTL?", "Save control to file?"="Save control to file?", "ignore empty fields?"="ignore empty fields?", "which axis?"="Row or Col?", "# index\nfor the text"="RowCol_index_All", "# index for\nthe values"="RowCol_index_ForRing", "Select the new type"="Select the new type", "append new data to control?"="AppendNewDataToControl?") -> (w253:T8)
        n110 = call "CC_CreateNewCTL.vi"("Error In"=w249, "Settings"=w253, "Save Path"="Single Control Save Path", "Clipboard Data"="Clipboard Data") -> ("Error Out"=w250:errorcluster)  [unwired: 7 in]
        n111 = call <vilib>:"Add State(s) to Queue__jki_lib_state_machine.vi"("State(s) in (\"\")"=w257) -> ("States Out"=w256:string)  [unwired: 14 in]
      }
      frame "CC: BatchNewControl" {
        n112 = call <vilib>:"Check if File or Folder Exists.vi"("error in (no error)"=w270, "path"="Batch_OutputFolder") -> ("error out"=w269:errorcluster, "file or folder exists?"=w265:bool, "dup path"=w266:path)  [unwired: 7 in]
        n113 = case shown="True" w265 {
          tunnel: w269 -> [w295 w296]
          tunnel: [w294 w296] -> w268
          tunnel: w266 -> [w293 _]
          frame False {
            n114 = Create Folder(path (use dialog)=w293, error in=w295) -> (error out=w294:errorcluster)  [unwired: 1 in, 2 out]
          }
          frame True {
          }
        }
        n115 = case shown="\"custom name\"" "Filename of new control" {
          tunnel: [TRUE ("s") FALSE ("s")] -> w284
          frame "unchanged", Default {
          }
          frame "custom name" {
          }
        }
        n116 = call <userlib>:"List Directory Recursive__ogtk.vi"("error in (no error)"=w268, "Treat llb files as directories? (FALSE)"=FALSE ("Treat LLBs as Folders?"), "pattern"="*.csv; *.txt", "Path"="Batch_InputFolder") -> ("error out"=w275:errorcluster, "file paths"=w274:path[])  [unwired: 4 in, 2 out]
        n117 = for {
          tunnel: "Batch_OutputFolder" -> [w337]
          shift-right: [w302] -> w290
          shift-left: w275 -> [w319]
          tunnel: w274 -> [w318] mode=indexing
          tunnel: "NewCTL_Open?" -> [w335]
          tunnel: "Batch_NewCTL_custom name" -> [w334]
          tunnel: "Batch_ignore empty fields?" -> [w331]
          tunnel: w284 -> [w330]
          tunnel: "NewCTLFile_AddPrefix?" -> [w328]
          tunnel: "NewCTLFile_AddSuffix?" -> [w324]
          tunnel: "prefix" -> [w322]
          tunnel: "suffix" -> [w321]
          tunnel: "BatchSelect the new type" -> [w315]
          tunnel: "Batch_RowCol_index_ForRing" -> [w314]
          tunnel: "Batch_RowCol_index_All" -> [w313]
          tunnel: "Batch_Row or Col?" -> [w312]
          tunnel: [w305] -> w264
          tunnel: "delimiter ('\\t', '\\s', ',')" -> [w300]
          tunnel: "file format (%.3f, %s, %d)" -> [w299]
          i -> [w305]
          stop <- w303 stop-if-true
          n118 = call <vilib>:"Get File Extension.vi"("error in (no error)"=w319, "file"=w318) -> ("error out"=w308:errorcluster, "filename without extension"=w317:string, "dup file"=w309:path)  [unwired: 5 in, 2 out]
          n119 = Number To Decimal String(number=w305) -> (decimal integer string=w333:string)  [unwired: 1 in]
          n120 = Concatenate Strings(w334, w333) -> (w332:string)
          n121 = Select(t=w321, s=w324, f="") -> (s? t:f=w323:string)
          n122 = Select(t=w322, s=w328, f="") -> (s? t:f=w326:string)
          n123 = Select(t=w317, s=w330, f=w332) -> (s? t:f=w329:string)
          n124 = Bundle By Name(cluster=T8 {"Save control to file?"=FALSE, "ignore empty fields?"=FALSE, "# index\nfor the text"=0, "# index for\nthe values"=0, "Select the new type"=enum."Array", "which axis?"=enum."Row", "append new data to control?"=enum."discard", "open new control?"=FALSE} ("Settings"), "Save control to file?"=TRUE, "open new control?"=w335, "ignore empty fields?"=w331, "which axis?"=w312, "# index\nfor the text"=w313, "# index for\nthe values"=w314, "Select the new type"=w315, "append new data to control?"=enum32{"discard", "top", "bottom"}."discard") -> (w338:T8)
          n125 = Concatenate Strings(w326, w329, w323, ".ctl" ("string")) -> (w320:string)
          n126 = call-poly <vilib>:"Read Delimited Spreadsheet.vi"("file path (dialog if empty)"=w309, "format (%s)"=w299, "error in (no error)"=w308, "delimiter (\\t)"=w300) -> ("new file path (Not A Path if cancelled)"=w304:path, "all rows"=w306:string[][], "error out"=w307:errorcluster)  [unwired: 6 in, 3 out]
          n127 = Build Path(base path=w337, name or relative path=w320) -> (appended path=w336:path)
          n128 = call "CC_CreateNewCTL.vi"("Error In"=w307, "Settings"=w338, "Save Path"=w336, "Clipboard Data"=w306) -> ("Error Out"=w303:errorcluster)  [unwired: 7 in]
          n129 = Strip Path(path=w304) -> (name=w301:string)  [unwired: 1 out]
          n130 = case shown="Error" w303 {
            selector: w303 -> [w340 w349]
            tunnel: [w340 w348] -> w302
            tunnel: w301 -> [_ w342]
            frame No Error {
            }
            frame Error {
              w341 = "\r"
              n131 = Unbundle(w349) -> ("status"=w347:bool, "code"=w346:i32, "source"=w345:string)
              n132 = Concatenate Strings(w345, w341, w341, "current File in progress: " ("string"), w341, w342) -> (w344:string)
              n133 = Bundle("status"=w347, "code"=w346, w344) -> (w348:cluster{"status":bool, "code":i32, string})  [unwired: 1 in]
            }
          }
        }
        n134 = Increment(x=w264) -> (x+1=w263:i32)
        n135 = Number To Decimal String(number=w263) -> (decimal integer string=w262:string)  [unwired: 1 in]
        n136 = call <vilib>:"Add State(s) to Queue__jki_lib_state_machine.vi"("State(s) in (\"\")"=w292) -> ("States Out"=w291:string)  [unwired: 14 in]
        n137 = Concatenate Strings(w262, " files processed" ("string")) -> (→"Batch_Status":string)
      }
      frame "PLM: SaveSinglePalette" {
      }
      frame "PLM: NewItemIcon" {
        n138 = call <vilib>:"Launch Icon Editor.vi"("error in (no error)"=w360, "Icon in"=refnum<class "Icon.lvclass"> refnum) -> ("error out"=w362:errorcluster, "Icon out"=w359:refnum<class "Icon.lvclass">)  [unwired: 7 in, 1 out]
        n139 = call <vilib>:"Get Flattened Image.vi"("error in (no error)"=w362, "lv_icon.lvlib:Icon.lvclass in"=w359) -> ("error out"=w361:errorcluster, "BW Image"=w356:T11, "Color Image"=w357:T11)  [unwired: 6 in, 1 out]
        n140 = call <vilib>:"Draw Flattened Pixmap.vi"("image data"=w357) -> ()  [unwired: 8 in, 1 out]
        n141 = call <vilib>:"Draw Flattened Pixmap.vi"("image data"=w356) -> ()  [unwired: 8 in, 1 out]
        n142 = call <vilib>:"Add State(s) to Queue__jki_lib_state_machine.vi"("State(s) in (\"\")"=w354, "State(s) at Back (\"\")"="PLM: UpdateImages" ("State(s) at Back (\"\")")) -> ("States Out"=w355:string)  [unwired: 13 in]
      }
      frame "PLM: LoadIconFromFile" {
        n143 = case shown="True" TRUE {
          tunnel: [w372 w375] -> w370
          tunnel: w369 -> [w372 w374]
          tunnel: [_ w373] -> w364
          frame False {
          }
          frame True {
            n144 = disable-structure shown="Disabled" {
              disable-tunnel: [w378 _] -> w375
              disable-tunnel: w374 -> [w377 _]
              disable-tunnel: [w376 _] -> w373
              frame Disabled {
                n145 = call "LoadAnyImage.vi"("Error In"=w377) -> ("Error Out"=w378:errorcluster, "Load Pic"=w376:picture)  [unwired: 9 in]
              }
              frame Enabled {
              }
            }
          }
        }
        n146 = call <vilib>:"Draw Flattened Pixmap.vi"("picture"=w364) -> ()  [unwired: 8 in, 1 out]
        n147 = call <vilib>:"Draw Flattened Pixmap.vi"("picture"=w364) -> ()  [unwired: 8 in, 1 out]
        n148 = call <vilib>:"Add State(s) to Queue__jki_lib_state_machine.vi"("State(s) in (\"\")"=w366, "State(s) at Back (\"\")"="PLM: UpdateImages" ("State(s) at Back (\"\")")) -> ("States Out"=w367:string)  [unwired: 13 in]
      }
      frame "PLM: UpdateImages" {
        n149 = disable-structure shown="Enabled" {
          disable-tunnel: w384 -> [w386 w387]
          disable-tunnel: [w385 w387] -> w383
          frame Disabled {
            n150 = Bundle By Name(cluster=w386) -> (w385:T9)  [unwired: 2 in]
          }
          frame Enabled {
          }
        }
        n151 = call <vilib>:"Add State(s) to Queue__jki_lib_state_machine.vi"("State(s) in (\"\")"=w380, "State(s) at Back (\"\")"="PLM: DrawPalImage" ("State(s) at Back (\"\")")) -> ("States Out"=w381:string)  [unwired: 13 in]
      }
      frame "PLM: Pal_New_Add" {
        n152 = call <vilib>:"Add State(s) to Queue__jki_lib_state_machine.vi"("State(s) in (\"\")"=w390, "State(s) at Back (\"\")"="PLM: DrawPalImage" ("State(s) at Back (\"\")")) -> ("States Out"=w391:string)  [unwired: 13 in]
      }
      frame "PLM: DrawPalImage" {
      }
    }
  }
